vi "Read.vi"(8 "error in (no error)":errorcluster, 11 "Simulation in":refnum<class "Simulation.lvclass">) -> (0 "error out":errorcluster, 2 "Message":string, 3 "Simulation out":refnum<class "Simulation.lvclass">)   [LabVIEW 2021, in "Simulation.lvclass"]
uses:
  Simulation.lvclass
  Simulation.lvclass/Simulation.ctl
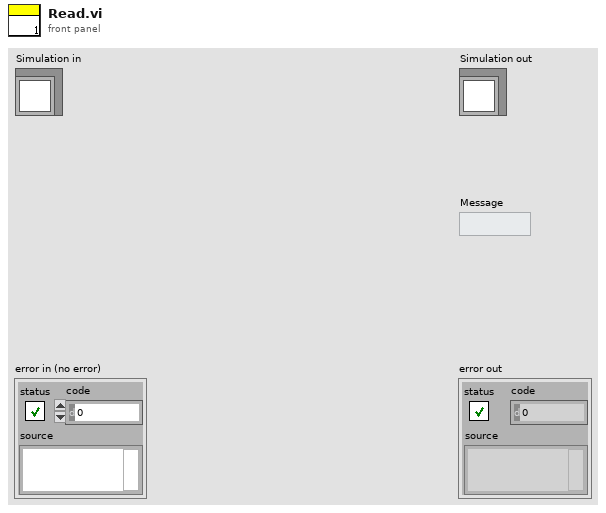
[diagram p1: front panel]
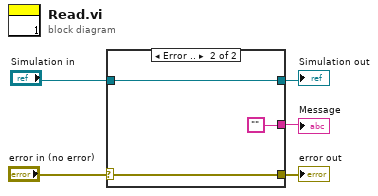
[diagram p0: block diagram]
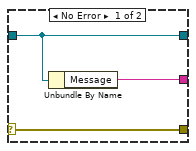
[diagram p2: hidden frame]
diagram:
  n1 = case shown="Error .." "error in (no error)" {
    selector: "error in (no error)" -> [w6 w9]
    tunnel: [w8 w11] -> w4
    tunnel: "Simulation in" -> [w8 w11]
    tunnel: [w7 ""] -> w2
    tunnel: [w6 w9] -> w1
    frame No Error {
      n2 = Unbundle By Name(w8) -> ("Message"=w7:string)
    }
    frame Error {
    }
  }
  "error out" <- w1
  "Simulation out" <- w4
  "Message" <- w2
